vi "Measurement UI.vi"() -> ()   [LabVIEW 2020, in "IVI Scope Measurement.lvlib"]
uses:
  IVI Scope Measurement.lvlib
panel:
  out "Waveform Array":dbl[](array[numeric])
  out "Waveform Graph":T1(graph)
  out "dt":dbl
  out "t0":dbl
  in  "Vertical Coupling":u32(ring)=1 items=["AC", "DC", "GND"]
  in  "Probe Attenuation":dbl=1.0
  in  "Vertical Offset":dbl=10.0
  in  "Vertical Range":dbl
  in  "Trigger Level":dbl
  in  "Minimum Record Length":i32
  in  "Time Per Record":dbl
  in  "Pin Name":string(combo)
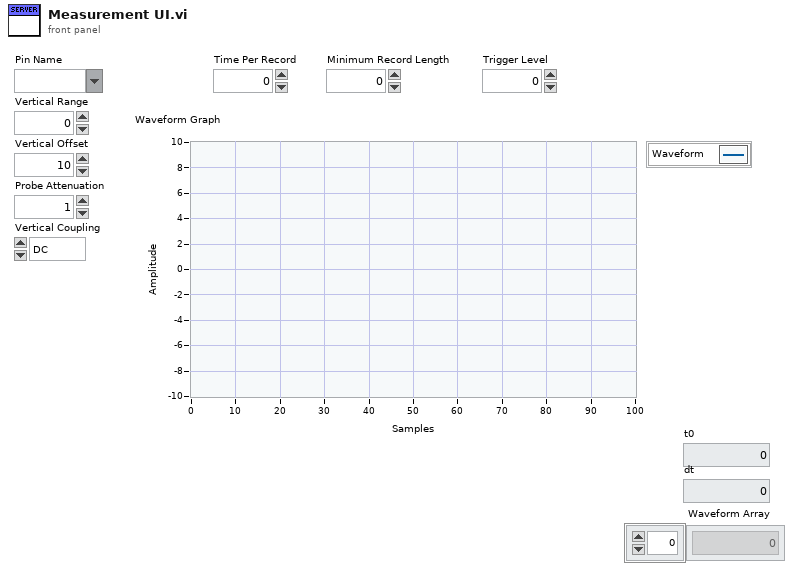
[diagram p1: front panel]
types:
  T1 = cluster{"t0":dbl, "dt":dbl, "Waveform Array":dbl[]}
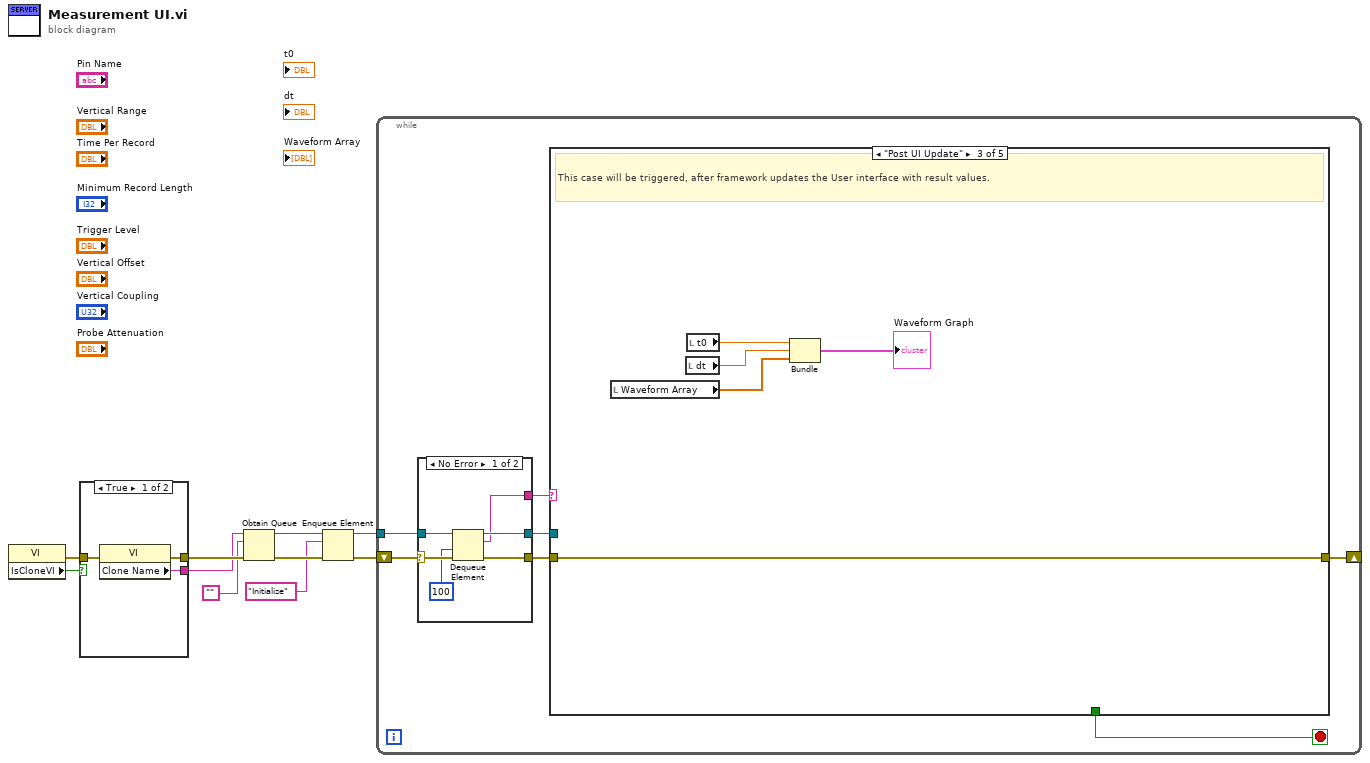
[diagram p0: block diagram]
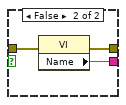
[diagram p2: hidden frame]
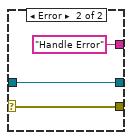
[diagram p3: hidden frame]
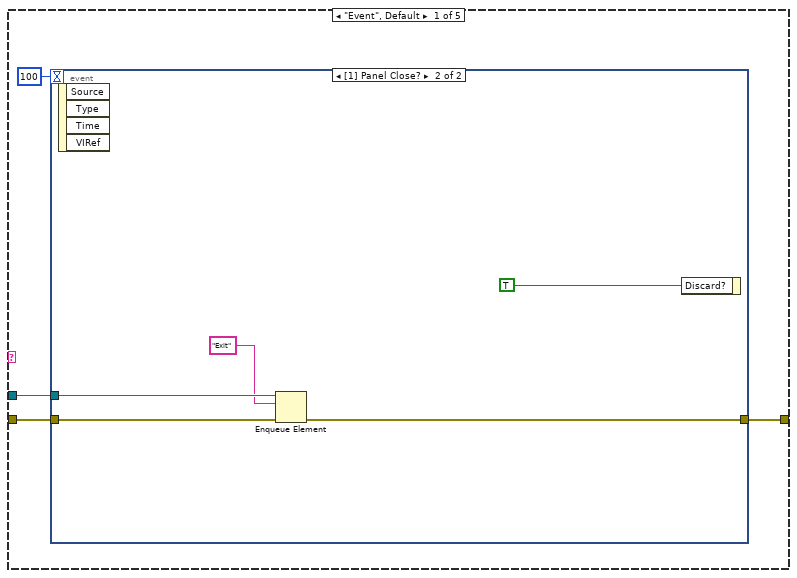
[diagram p4: hidden frame]
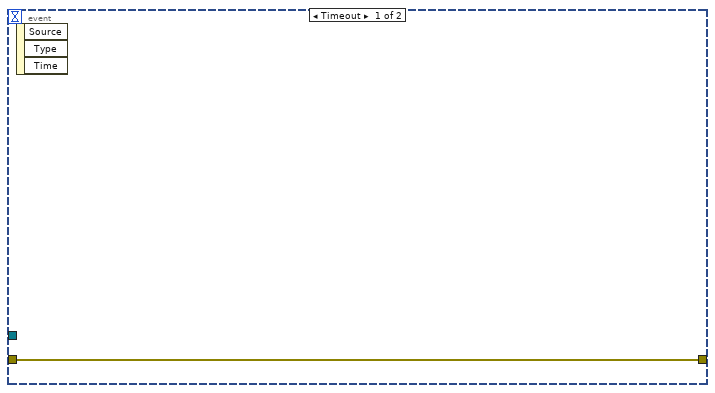
[diagram p5: hidden frame]
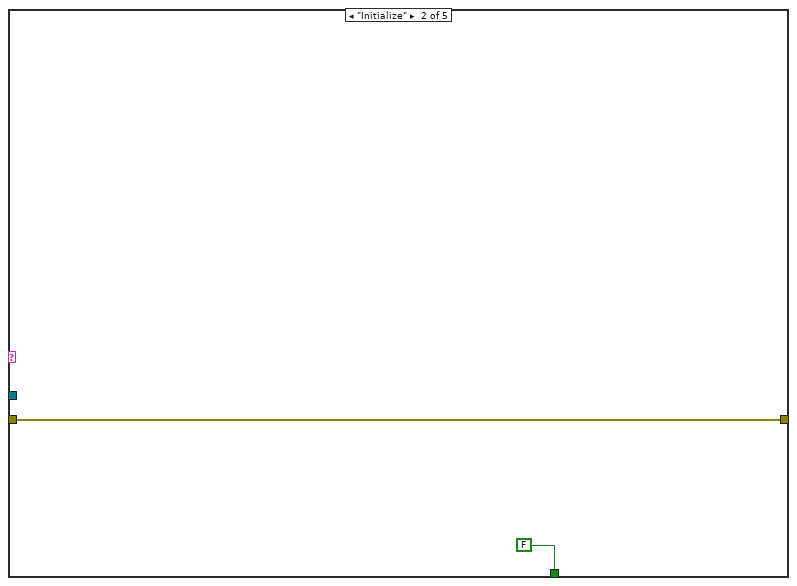
[diagram p6: hidden frame]
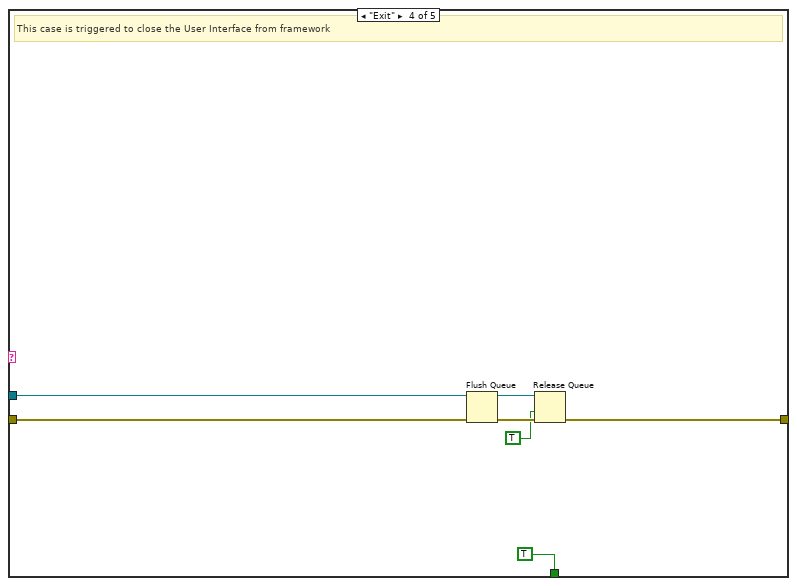
[diagram p7: hidden frame]
diagram:
  n1 = property class="VI"() -> (error out=w1:errorcluster, "IsCloneVI"=w2:bool)  [unwired: 2 in, 1 out]
  n2 = case shown="True" w2 {
    tunnel: [w13 w16] -> w10
    tunnel: [w12 w15] -> w9
    tunnel: w1 -> [w11 w14]
    frame True {
      n3 = property class="VI"(error in=w11) -> (error out=w13:errorcluster, "Clone Name"=w12:string)  [unwired: 1 in, 1 out]
    }
    frame False {
      n4 = property class="VI"(error in=w14) -> (error out=w16:errorcluster, "Name"=w15:string)  [unwired: 1 in, 1 out]
    }
  }
  n5 = Obtain Queue(name (unnamed)=w9, element data type="", error in (no error)=w10) -> (queue out=w6:refnum<queue>, error out=w8:errorcluster)  [unwired: 2 in, 1 out]
  n6 = Enqueue Element(queue=w6, element="Initialize", error in (no error)=w8) -> (queue out=w5:refnum<queue>, error out=w7:errorcluster)  [unwired: 1 in, 1 out]
  n7 = while {
    shift-right: [w18] -> _
    shift-left: w7 -> [w23]
    tunnel: w5 -> [w21]
    stop <- w17 stop-if-true
    n8 = case shown="No Error" w23 {
      selector: w23 -> [w29 w32]
      tunnel: [w28 w32] -> w22
      tunnel: w21 -> [w27 w31]
      tunnel: [w26 w31] -> w20
      tunnel: [w25 "Handle Error"] -> w19
      frame No Error {
        n9 = Dequeue Element(queue=w27, timeout in ms (-1)=100, error in (no error)=w29) -> (queue out=w26:refnum<queue>, element=w25:string, error out=w28:errorcluster)  [unwired: 1 out]
      }
      frame Error {
      }
    }
    n10 = case shown="\"Post UI Update\"" w19 {
      tunnel: w22 -> [w35 w44 w49 w56 w57]
      tunnel: w20 -> [w33 _ _ w54 _]
      tunnel: [w36 w44 w49 w51 w57] -> w18
      tunnel: [_ FALSE _ TRUE _] -> w17
      frame "Event", Default {
        n11 = event shown="[1] Panel Close?" {
          selector: _ -> [_ _]
          dyn-events: _ -> [_ _]
          timeout: 100 -> [_ _]
          tunnel: [w37 w40] -> w36
          tunnel: w35 -> [w37 w41]
          tunnel: w33 -> [_ w39]
          event Timeout {
            n12 = event-data() -> ()  [unwired: 1 in, 3 out]
          }
          event Panel Close? {
            n13 = event-data() -> ()  [unwired: 1 in, 4 out]
            n14 = Enqueue Element(queue=w39, element="Exit", error in (no error)=w41) -> (error out=w40:errorcluster)  [unwired: 1 in, 2 out]
            n15 = event-data("Discard?"=TRUE) -> ()  [unwired: 1 in, 1 out]
          }
        }
      }
      frame "Initialize" {
      }
      frame "Post UI Update" {
        # "This case will be triggered, after framework updates the User interface with result values."
        n16 = local read "Waveform Array"() -> (w46:dbl[])
        n17 = local read "dt"() -> (w47:dbl)
        n18 = local read "t0"() -> (w48:dbl)
        n19 = Bundle("t0"=w48, "dt"=w47, "Waveform Array"=w46) -> (→"Waveform Graph":T1)  [unwired: 1 out]
      }
      frame "Exit" {
        # "This case is triggered to close the User Interface from framework"
        n20 = Flush Queue(queue=w54, error in (no error)=w56) -> (queue out=w53:refnum<queue>, error out=w52:errorcluster)  [unwired: 1 out]
        n21 = Release Queue(queue=w53, force destroy? (F)=TRUE, error in (no error)=w52) -> (error out=w51:errorcluster)  [unwired: 2 out]
      }
      frame "Handle Error" {
      }
    }
  }
